vi "GM Test Pulse Generator.vi"() -> ()   [LabVIEW 2010]
uses:
  <vilib>/DAQmx/write.llb/DAQmx Write (Analog DBL 1Chan 1Samp).vi
  <vilib>/DAQmx/create/channels.llb/DAQmx Create Channel (AO-Voltage-Basic).vi
  <vilib>/DAQmx/configure/timing.llb/DAQmx Timing (Sample Clock).vi
  <vilib>/daqmx/miscellaneous.llb/DAQmx Fill In Error Info.vi
panel:
  in  "Decay Constant":dbl=500.0
  in  "Pulse Height (V)":dbl=-0.04
  in  "Milliseconds between pulses":u32=5
  in  "stop":bool
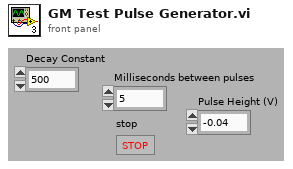
[diagram p1: front panel]
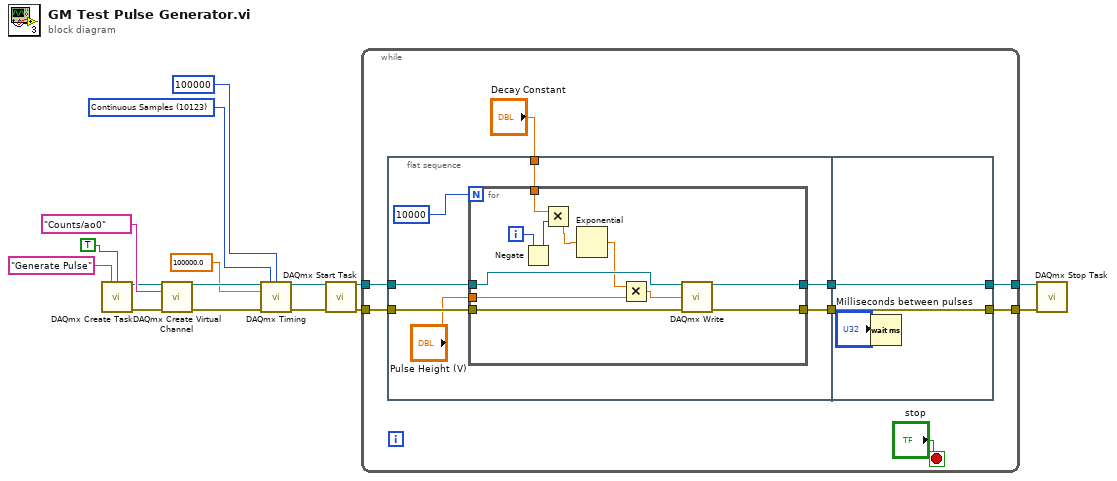
[diagram p0: block diagram]
diagram:
  w11 = 10123 items=["Finite Samples"=10178, "Continuous Samples"=10123, "Hardware Timed Single Point"=12522] ("sample mode")
  n1 = call <vilib>:"DAQmx Create Task.vi"("new task name"="Generate Pulse", "auto cleanup"=TRUE) -> ("task out"=w13:refnum<k21>, "error out"=w12:errorcluster)  [unwired: 12 in]
  n2 = call-poly <vilib>:"DAQmx Create Virtual Channel.vi"("task in"=w13, "physical channels"=tag "Counts/ao0", "error in"=w12) -> ("task out"=w10:refnum<k21>, "error out"=w9:errorcluster)  [unwired: 11 in]
  n3 = call-poly <vilib>:"DAQmx Timing.vi"("task/channels in"=w10, "sample mode"=w11, "samples per channel"=100000, "rate"=100000.0 ("Sample Clock Rate (Hz)"), "error in"=w9) -> ("task out"=w8:refnum<k21>, "error out"=w6:errorcluster)  [unwired: 9 in]
  n4 = call <vilib>:"DAQmx Start Task.vi"("task/channels in"=w8, "error in"=w6) -> ("task out"=w7:refnum<k21>, "error out"=w5:errorcluster)  [unwired: 12 in]
  n5 = while {
    tunnel: w7 -> [w24]
    tunnel: w5 -> [w23]
    tunnel: [w21] -> w2
    tunnel: [w20] -> w1
    stop <- "stop" stop-if-true
    n6 = flat-sequence {
      tunnel: w24 -> [w31]
      tunnel: w23 -> [w30]
      tunnel: [w28] -> w19
      tunnel: [w27] -> w18
      tunnel: "Decay Constant" -> [w25]
      tunnel: [w44] -> w20
      tunnel: [w45] -> w21
      tunnel: w19 -> [w44]
      tunnel: w18 -> [w45]
      frame #0 {
        n7 = for {
          N: 10000 -> [_]
          tunnel: w31 -> [w42]
          tunnel: w30 -> [w41]
          tunnel: "Pulse Height (V)" -> [w32]
          tunnel: [w39] -> w28
          tunnel: [w38] -> w27
          tunnel: w25 -> [w36]
          i -> [w37]
          n8 = Negate(x=w37) -> (-x=w35:i32)
          n9 = Multiply(x=w36, y=w35) -> (x*y=w34:dbl)
          n10 = Exponential(1:w34) -> (0:w33:dbl)
          n11 = Multiply(x=w33, y=w32) -> (x*y=w40:dbl)
          n12 = call-poly <vilib>:"DAQmx Write.vi"("task/channels in"=w42, "data"=w40, "error in"=w41) -> ("task out"=w38:refnum<k21>, "error out"=w39:errorcluster)  [unwired: 10 in, 1 out]
        }
      }
      frame #1 {
        n13 = Wait (ms)(milliseconds to wait="Milliseconds between pulses") -> ()  [unwired: 1 out]
      }
    }
  }
  n14 = call <vilib>:"DAQmx Stop Task.vi"("task/channels in"=w2, "error in"=w1) -> ()  [unwired: 12 in, 2 out]
